vi "Calc_Sharpness_Metric_SLM.vi"(10 "AC Image":dbl[][](array[numeric]), 11 "Numeric in":dbl) -> (3 "Numeric out":dbl)   [LabVIEW 2018]
uses:
  <vilib>/Analysis/2dsp.llb/2D Real FFT.vi
  <vilib>/Analysis/NI_AALPro.lvlib
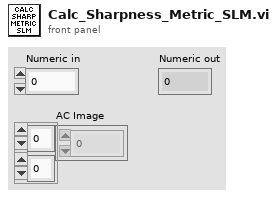
[diagram p1: front panel]
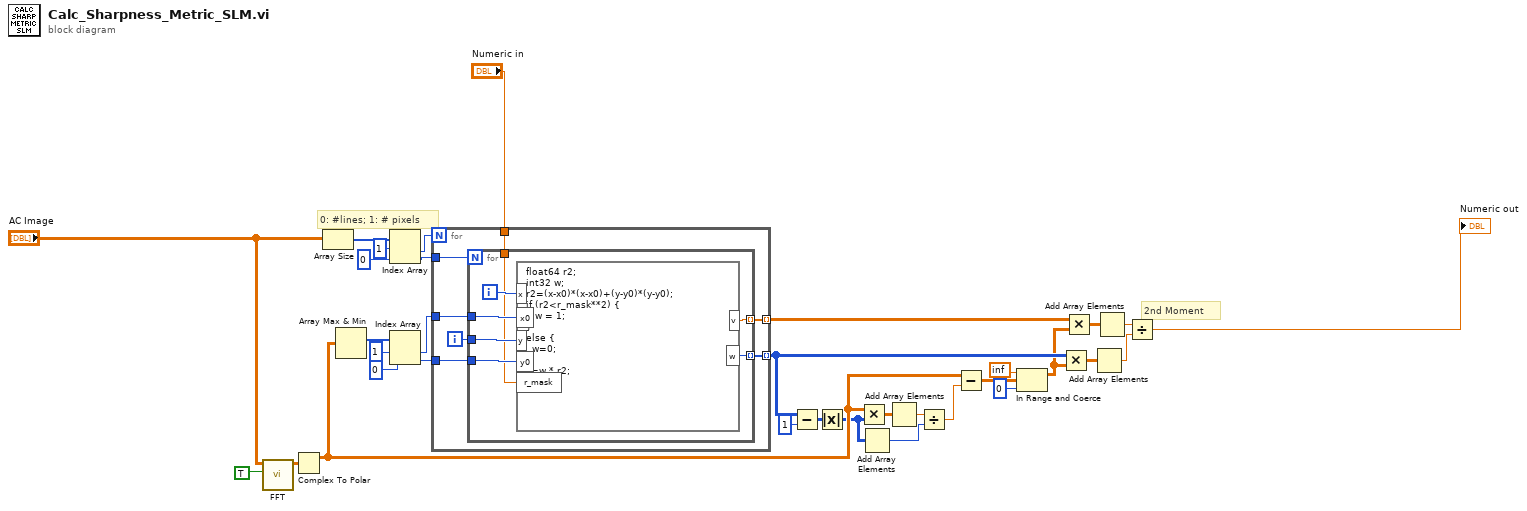
[diagram p0: block diagram]
diagram:
  # "2nd Moment"
  # "0: #lines; 1: # pixels"
  n1 = call-poly <vilib>:"FFT.vi"("shift?"=TRUE, "X"="AC Image") -> ("FFT {X}"=w2:cdb[][])  [unwired: 2 in, 7 out]
  n2 = Complex To Polar(r * e^(i*theta)=w2) -> (r=w29:dbl[][])  [unwired: 1 out]
  n3 = Array Size(array="AC Image") -> (size(s)=w16:i32[])
  n4 = Array Max & Min(array=w29) -> (max index (indices)=w3:i32[])  [unwired: 3 out]
  n5 = Index Array(array=w16, index #1=1 ("index"), index #2=0 ("index")) -> (element #1=w19:i32, element #2=w18:i32)
  n6 = Index Array(array=w3, index #1=1 ("index"), index #2=0 ("index")) -> (element #1=w6:i32, element #2=w7:i32)
  n7 = for {
    N: w19 -> [_]
    tunnel: w18 -> [w40]
    tunnel: w6 -> [w39]
    tunnel: w7 -> [w38]
    tunnel: [w37] -> w8 mode=indexing
    tunnel: [w35] -> w28 mode=indexing
    tunnel: "Numeric in" -> [w34]
    i -> [w36]
    n8 = for {
      N: w40 -> [_]
      tunnel: w39 -> [w45]
      tunnel: w38 -> [w43]
      tunnel: [w47] -> w37 mode=indexing
      tunnel: w36 -> [w44]
      tunnel: [w42] -> w35 mode=indexing
      tunnel: w34 -> [w41]
      i -> [w46]
      n9 = formula code="float64 r2;\nint32 w;\nr2=(x-x0)*(x-x0)+(y-y0)*(y-y0);\nif (r2<r_mask**2) {\n   w = 1;\n}\nelse {\n  w=0;\n}\nv=w * r2;"("x"=w46, "x0"=w45, "y"=w44, "y0"=w43, "r_mask"=w41) -> ("v"=w47:dbl, "w"=w42:i32)
    }
  }
  n10 = Subtract(x=w28, y=i8 1) -> (x-y=w22:i32[][])
  n11 = Absolute Value(x=w22) -> (abs(x)=w27:i32[][])
  n12 = Multiply(x=w29, y=w27) -> (x*y=w24:dbl[][])
  n13 = Add Array Elements(numeric array=w27) -> (sum=w26:i32)
  n14 = Add Array Elements(numeric array=w24) -> (sum=w25:dbl)
  n15 = Divide(x=w25, y=w26) -> (x/y=w32:dbl)
  n16 = Subtract(x=w29, y=w32) -> (x-y=w13:dbl[][])
  n17 = In Range and Coerce(upper limit=inf, x=w13, lower limit=0) -> (coerced(x)=w23:dbl[][])  [unwired: 1 out]
  n18 = Multiply(x=w28, y=w23) -> (x*y=w20:dbl[][])
  n19 = Multiply(x=w8, y=w23) -> (x*y=w9:dbl[][])
  n20 = Add Array Elements(numeric array=w20) -> (sum=w10:dbl)
  n21 = Add Array Elements(numeric array=w9) -> (sum=w11:dbl)
  n22 = Divide(x=w11, y=w10) -> (x/y=→"Numeric out":dbl)
